vi "SPI API FPGA.vi"() -> ()   [LabVIEW 2014]
uses:
  <userlib>/_NI SPI IP/FPGA/Controllers/Public/Transfer Settings.ctl
  <vilib>/Platform/TimedLoop/XDataNode/timing_clust.ctl
  <vilib>/Platform/TimedLoop/XDataNode/nitl_modes.ctl
  <vilib>/Platform/TimedLoop/XDataNode/wakeup.ctl
  <vilib>/SPI API/SPIAPI/DIO/SPI Digital IO Lines.ctl
  <vilib>/rvi/Emulation/niFpgaGetClockAttributes.vi
  <vilib>/rvi/Emulation/niFpgaSctlEmulationGetInTimedLoop.vi
  <vilib>/rvi/Emulation/niFpgaEmulationReportErrorSimple.vi
  <vilib>/rvi/Emulation/niFpgaCriticalErrorInLSC.vi
  <vilib>/rvi/interface/RandomDataEmulation/niFpgaRandomDataHandleErrors.vi
  <vilib>/Platform/TimedLoop/XDataNode/XDataNode.xnode
  <vilib>/rvi/DataTransferAndStorage/Container/XNode/niFpgaContainer.xnode
  <vilib>/rvi/interface/RandomDataEmulation/nirviRandomDataFpgaReadWriteTemplate.vi
  <vilib>/Platform/TimedLoop/XDataNode/XDNodeRunTimeDep.lvlib
  <userlib>/_NI SPI IP/FPGA/Controllers/NI SPI IP FPGA.lvlib
panel:
  out "Chip Select":u8
  out "Data to DAC":u64
  out "FPGA Error":errorcluster
  out "Actual Loop Ticks":u32
  in  "SPI PHY Settings":T1={"Divide Value"=20, "Transfer Length (bits)"=32, "CS Asserted Polarity"=FALSE, "Clock Polarity (CPOL)"=FALSE, "Clock Phase (CPHA)"=FALSE, "Lengthen MISO Setup"=FALSE, "Direction Change Bit"=0, "MOSI Starts as Output"=FALSE, "Tristatable MOSI"=FALSE} {"Direction Change Bit" max=64 step=1; "Transfer Length (bits)" min=1 max=64 step=1}
  out "read Iterations":i32
  out "NC":u64
  out "oclk div":u32
  out "oclk freq":u32
  in  "Sample Rate (S/s)":u32=10000
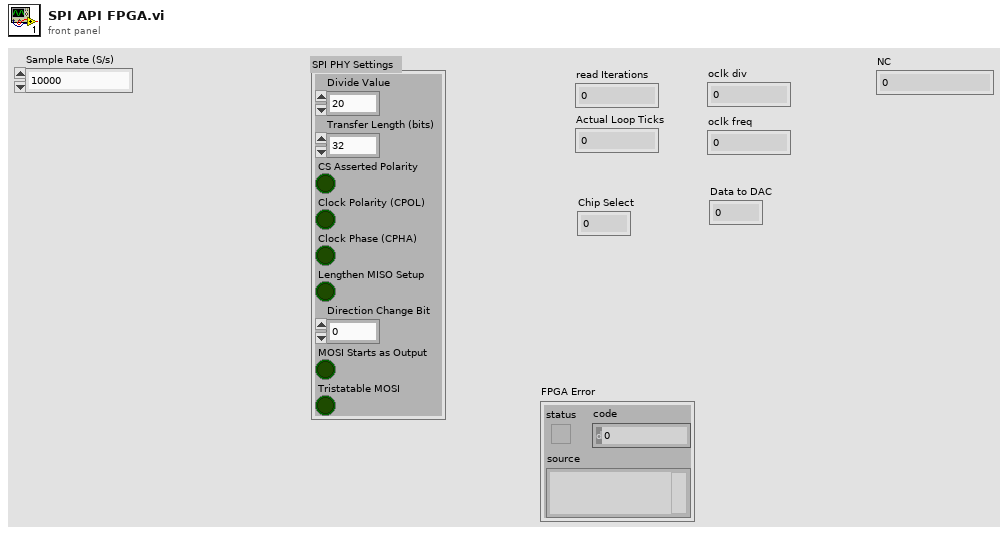
[diagram p1: front panel]
types:
  T1 = typedef "NI SPI IP FPGA.lvlib/Transfer Settings.ctl" = cluster{"Divide Value":u8, "Transfer Length (bits)":u8, "CS Asserted Polarity":bool, "Clock Polarity (CPOL)":bool, "Clock Phase (CPHA)":bool, "Lengthen MISO Setup":bool, "Direction Change Bit":u8, "MOSI Starts as Output":bool, "Tristatable MOSI":bool}
  T2 = typedef "SPI Digital IO Lines.ctl" = cluster{"SCLK":refnum<k21>, "MISO":refnum<k21>, "MOSI":refnum<k21>, "CS 0":refnum<k21>, "CS 1":refnum<k21>, "CS 2":refnum<k21>, "CS 3":refnum<k21>, "CS 4":refnum<k21>, "CS 5":refnum<k21>}
  T3 = typedef "Internal Data (SPI API).ctl" = cluster{"DLU To SPI Engine Data FIFO":refnum<k21>, "SPI Engine to DLU Data FIFO":refnum<k21>, "Data to SPI Engine (Cache) Register":refnum<k21>, "SPI PHY Settings to SPI Engine (Cahche) Register":refnum<k21>}
  T4 = typedef "XDNodeRunTimeDep.lvlib/timing_clust.ctl" = cluster{"Expected End [f-1]":u64, "Actual End [f-1]":u64, "Finished Late? [f-1]":bool, "Expected End [i-1]":u64, "Actual End [i-1]":u64, "Finished Late? [i-1]":bool, "Expected Start [i]":u64, "Actual Start [i]":u64, "Expected Start [f]":u64, "Actual Start [f]":u64, "Source Name":string, "Structure Name":string, "Period":i64, "Deadline":i64, "Offset":i64, "Start":i64, "Priority":i32, "Timeout":i32, "Mode":T5, "Wakeup Reason":T6, "Error":errorcluster, "Source Type":string, "Secondary Source Type":string, "Global End Time":u64, "Global Start Time":u64, "Frame Duration":u64, "Iteration Duration":u64, "Assigned CPU":i32, "I/O Scan Engine Mode":u32}
  T5 = typedef "XDNodeRunTimeDep.lvlib/nitl_modes.ctl" = enum32{"No Change", "Process missed periods, maintain original phase", "Discard missed periods, maintain original phase", "Process missed periods, ignore original phase", "Discard missed periods, ignore original phase"}
  T6 = typedef "XDNodeRunTimeDep.lvlib/wakeup.ctl" = enum32{"Normal", "Aborted", "Asynchronous wakeup", "Timing source error", "Timed loop error", "Timeout"}
  T7 = typedef "SPI Response Information.ctl" = cluster{"Data to Node":u64, "Node Id":u16}
  T8 = typedef "NI SPI IP FPGA.lvlib/Spi Master Inputs.ctl" = cluster{"MISO":bool}
  T9 = typedef "NI SPI IP FPGA.lvlib/Spi Master Outputs.ctl" = cluster{"Chip Select":bool, "Clock":bool, "MOSI":bool, "MOSI OE":bool}
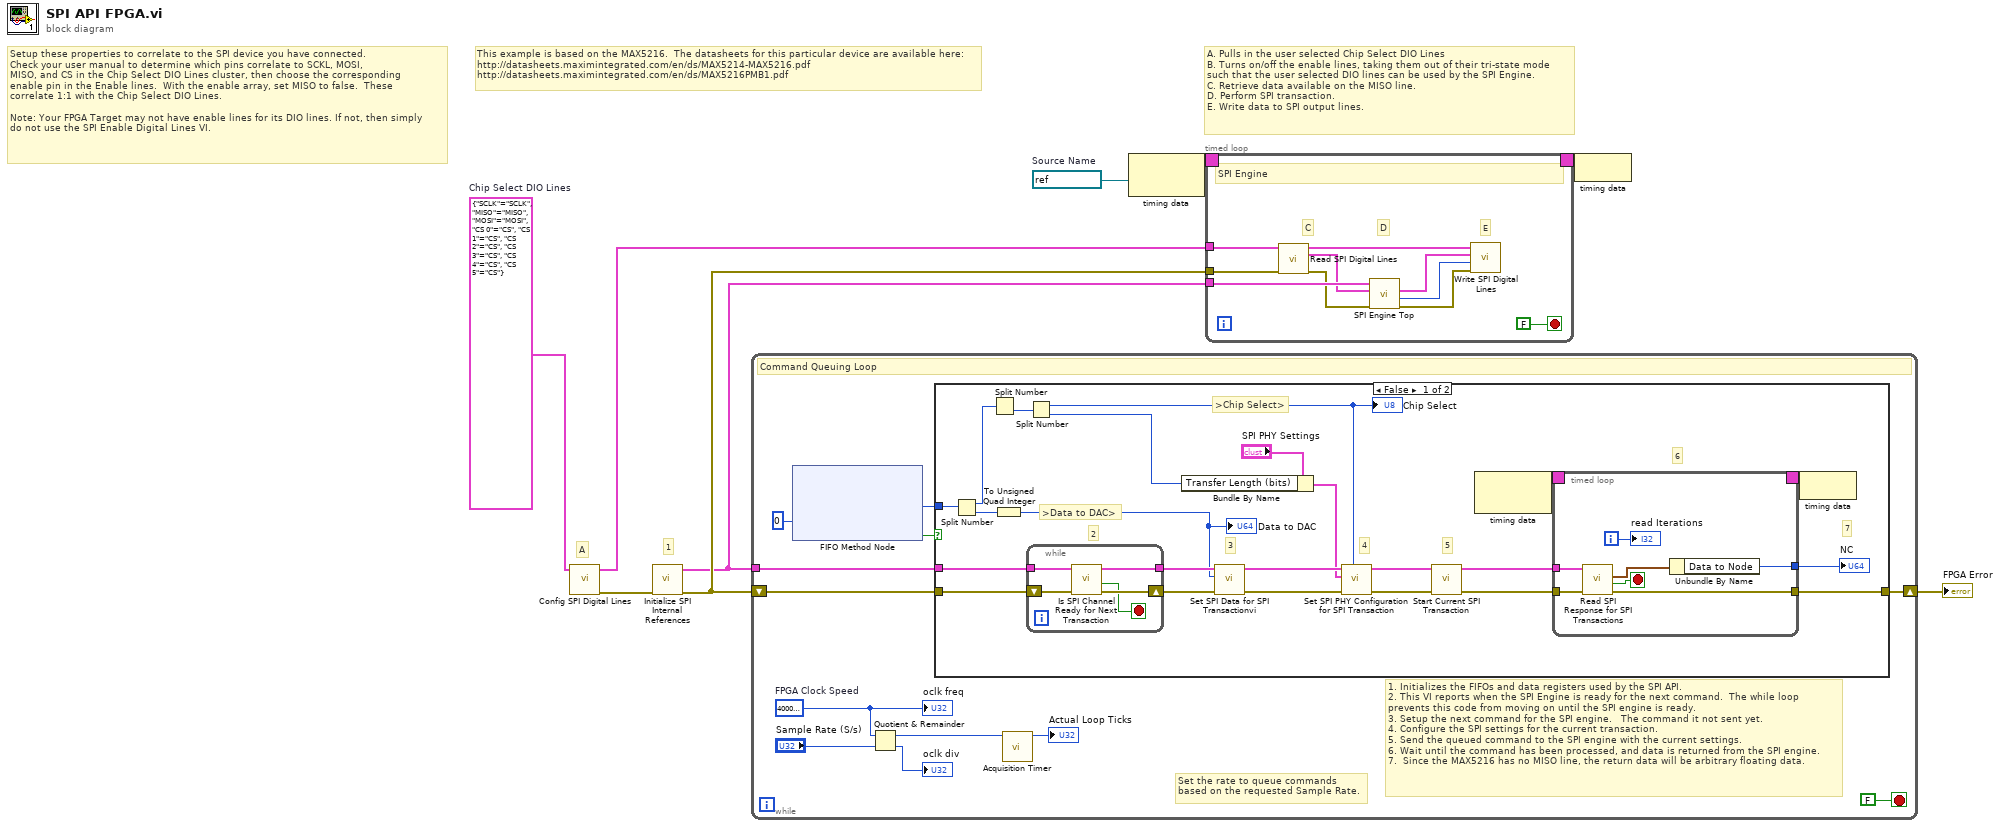
[diagram p0: block diagram]
diagram:
  w6 = T2 {"SCLK"="SCLK", "MISO"="MISO", "MOSI"="MOSI", "CS 0"="CS", "CS 1"="CS", "CS 2"="CS", "CS 3"="CS", "CS 4"="CS", "CS 5"="CS"}  # Chip Select DIO Lines
  w7 = refnum<k21> "120MHz"  # Source Name
  # "This example is based on the MAX5216.  The datasheets for this particular device are available here:\nhttp://datasheets.maximintegrated.com/en/ds/MAX5214-MAX5216.pdf\nhttp://datasheets.maximintegrated.com/en/ds/MAX5216PMB1.pdf"
  # "A. Pulls in the user selected Chip Select DIO Lines\nB. Turns on/off the enable lines, taking them out of their tri-state mode \nsuch that the user selected DIO lines can be used by the SPI Engine.\nC. Retrieve data available on the MISO line.\nD. Perform SPI transaction.\nE. Write data to SPI output lines."
  # "A"
  # "1"
  # "Setup these properties to correlate to the SPI device you have connected.\nCheck your user manual to determine which pins correlate to SCKL, MOSI,\nMISO, and CS in the Chip Select DIO Lines cluster, then choose the corresponding\nenable pin in the Enable lines.  With the enable array, set MISO to false.  These\ncorrelate 1:1 with the Chip Select DIO Lines.\n\nNote: Your FPGA Target may not have enable lines for its DIO lines. If not, then simply\ndo not use the SPI Enable Digital Lines VI."
  n1 = call <vilib>:"Config SPI Digital Lines.vi"("SPI DIO Lines"=w6) -> ("error out"=w2:errorcluster, "Chip Select DIO Lines"=w1:T2)  [unwired: 9 in]
  n2 = call <vilib>:"Initialize SPI Internal References.vi"("error in"=w2) -> ("error out"=w4:errorcluster, "SPI API References"=w3:T3)  [unwired: 9 in]
  n3 = while {
    shift-right: [w17] -> w5
    shift-left: w4 -> [w19]
    tunnel: w3 -> [w20]
    stop <- FALSE stop-if-true
    w16 = u32 40000000  # FPGA Clock Speed
    # "1. Initializes the FIFOs and data registers used by the SPI API.\n2. This VI reports when the SPI Engine is ready for the next command.  The while loop \nprevents this code from moving on until the SPI engine is ready.\n3. Setup the next command for the SPI engine.   The command it not sent yet.\n4. Configure the SPI settings for the current transaction.\n5. Send the queued command to the SPI engine with the current settings.\n6. Wait until the command has been processed, and data is returned from the SPI engine.\n7.  Since the MAX5216 has no MISO line, the return data will be arbitrary floating data."
    # "Set the rate to queue commands\nbased on the requested Sample Rate."
    # "Command Queuing Loop"
    n4 = xnode ("FIFO Method Node")("Timeout"=0) -> ("Element"=w12:u64, "Timed Out?"=w11:bool)  [unwired: 1 in, 1 out]
    n5 = Quotient & Remainder(x=w16, y="Sample Rate (S/s)") -> (x-y*floor(x/y)=w13:u32, floor(x/y)=→"oclk div":u32)
    n6 = case shown="False" w11 {
      tunnel: w20 -> [w40 _]
      tunnel: w19 -> [w39 w61]
      tunnel: [w32 w61] -> w17
      tunnel: w12 -> [w30 _]
      frame False {
        # ">Data to DAC>"
        # ">Chip Select>"
        # "7"
        # "6"
        # "5"
        # "4"
        # "3"
        # "2"
        n7 = Split Number(x=w30) -> (hi(x)=w28:u32, lo(x)=w29:u32)
        n8 = Split Number(x=w28) -> (lo(x)=w27:u16)  [unwired: 1 out]
        n9 = To Unsigned Quad Integer(1:w29) -> (0:w26:u64)
        "Data to DAC" <- w26
        n10 = Split Number(x=w27) -> (hi(x)=w22:u8, lo(x)=w23:u8)
        "Chip Select" <- w22
        n11 = while {
          shift-right: [w49] -> w42
          shift-left: w39 -> [w46]
          tunnel: w40 -> [w47]
          tunnel: [w48] -> w41
          stop <- w45 stop-if-true
          n12 = call <vilib>:"Is SPI Channel Ready for Next Transaction.vi"("error in"=w46, "Private Data In"=w47) -> ("error out"=w49:errorcluster, "SPI Channel Ready"=w45:bool, "Private Data Out"=w48:T3)  [unwired: 6 in, 1 out]
        }
        n13 = Bundle By Name(cluster="SPI PHY Settings", "Transfer Length (bits)"=w23) -> (w24:T1)
        n14 = call <vilib>:"Set SPI Data for SPI Transactionvi.vi"("error in"=w42, "Data In"=w26, "Private Data In"=w41) -> ("error out"=w36:errorcluster, "Private Data Out"=w37:T3)  [unwired: 7 in]
        n15 = call <vilib>:"Set SPI PHY Configuration for SPI Transaction.vi"("Chip Select"=w22, "error in"=w36, "SPI PHY Settings"=w24, "Private Data In"=w37) -> ("error out"=w34:errorcluster, "Private Data Out"=w35:T3)  [unwired: 6 in]
        n16 = call <vilib>:"Start Current SPI Transaction.vi"("error in"=w34, "Private Data In"=w35) -> ("error out"=w38:errorcluster, "Private Data Out"=w33:T3)  [unwired: 7 in, 1 out]
        n17 = node-c288() -> (w44:T4)  [unwired: 1 in]
        n18 = timed-loop {
          timing: w44 -> [_]
          timing-out: [_] -> w43
          tunnel: w38 -> [w56]
          tunnel: w33 -> [w55]
          tunnel: [w50] -> w31
          tunnel: [w52] -> w32
          i -> [w51]
          stop <- w54 stop-if-true
          n19 = call <vilib>:"Read SPI Response for SPI Transactions.vi"("error in"=w56, "Private Data In"=w55) -> ("error out"=w52:errorcluster, "Read Data Valid?"=w54:bool, "Read Data"=w53:T7)  [unwired: 6 in, 1 out]
          n20 = Unbundle By Name(w53) -> ("Data to Node"=w50:u64)
          "read Iterations" <- w51
        }
        "NC" <- w31
        n21 = node-c288(w43) -> ()
      }
      frame True {
      }
    }
    n22 = call <vilib>:"Acquisition Timer.vi"("Loop Time (Ticks)"=w13) -> ("Actual Time (Ticks)"=→"Actual Loop Ticks":u32)  [unwired: 10 in]
    "oclk freq" <- w16
  }
  "FPGA Error" <- w5
  n23 = node-c288(w7) -> (w9:T4)
  n24 = timed-loop {
    tunnel: w3 -> [w68]
    tunnel: w4 -> [w66]
    tunnel: w1 -> [w70]
    timing: w9 -> [_]
    timing-out: [_] -> w8
    stop <- FALSE stop-if-true
    # "E"
    # "D"
    # "C"
    # "SPI Engine"
    n25 = call <vilib>:"Read SPI Digital Lines.vi"("Chip Select DIO Lines"=w70, "error in"=w66) -> ("Chip Select DIO Lines Out"=w71:T2, "SPI Read Data"=w67:T8, "error out"=w65:errorcluster)  [unwired: 11 in]
    n26 = call <vilib>:"SPI Engine Top.vi"("error in"=w65, "SPI Read Data"=w67, "SPI API References"=w68) -> ("error out"=w64:errorcluster, "Chip Select ID"=w63:u8, "SPI DIO Output"=w69:T9)  [unwired: 5 in, 1 out]
    n27 = call <vilib>:"Write SPI Digital Lines.vi"("error in"=w64, "CS Index"=w63, "spi output"=w69, "Chip Select DIO Lines"=w71) -> ()  [unwired: 6 in, 2 out]
  }
  n28 = node-c288(w8) -> ()
